vi "tls http connection handler.vi"(8 "http responder":refnum<class "http responder.lvclass">, 9 "remote address":string, 10 "basic HTTP handler dataset":refnum<class "basic HTTP handler dataset.lvclass">, 11 "connection":refnum<k5>) -> ()   [LabVIEW 2016, in "TLS HTTP server.lvclass"]
uses:
  TLS HTTP server.lvclass
  HTTP responder/http responder.lvclass
  HTTP handler dataset/basic HTTP handler dataset.lvclass
  HTTP server/http request.ctl
  HTTP server/http method.ctl
  HTTP headers/http header data.ctl
  HTTP server/http response.ctl
  HTTP server/http response packet type.ctl
  TLS handler dataset/TLS HTTP handler dataset.lvclass
  HTTP handler dataset/basic HTTP handler dataset.lvclass/basic HTTP handler dataset.ctl
  HTTP server/http parse state.ctl
  HTTP server/Basic HTTP server.lvclass
  HTTP headers/http headers.lvlib
  lvlibtls/socket connection/lvlibretls connection.lvclass
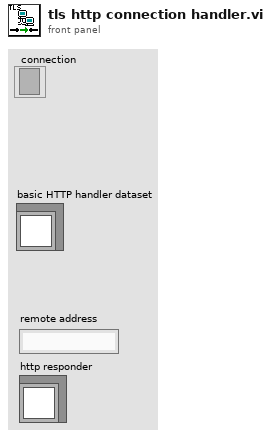
[diagram p1: front panel]
types:
  T1 = typedef "Basic HTTP server.lvclass/http response.ctl" = cluster{"packet type":T2, "reason code":u16, "status string":string, "headers":T3, "cookies":string[], "data":string}
  T2 = typedef "Basic HTTP server.lvclass/http response packet type.ctl" = enum16{"full response", "header only", "data only", "last data", "raw output"}
  T3 = typedef "http headers.lvlib/http header data.ctl" = cluster{"lookup":variant}
  T4 = typedef "Basic HTTP server.lvclass/http request.ctl" = cluster{"type":T5, "remote address":string, "method":string, "url":string, "version":string, "headers":T3, "data":string}
  T5 = typedef "Basic HTTP server.lvclass/http method.ctl" = enum16{"application", "error", "upgrade", "expect"}
  T6 = typedef "Basic HTTP server.lvclass/http server info.ctl" = cluster{"port":u16}
  T7 = typedef "Basic HTTP server.lvclass/http server properties.ctl" = cluster{"max url size":i32, "max header":i32, "timeout ms":i32, "max data size":i32}
  T8 = typedef "Basic HTTP server.lvclass/http parse state.ctl" = enum16{"function", "headers", "data"}
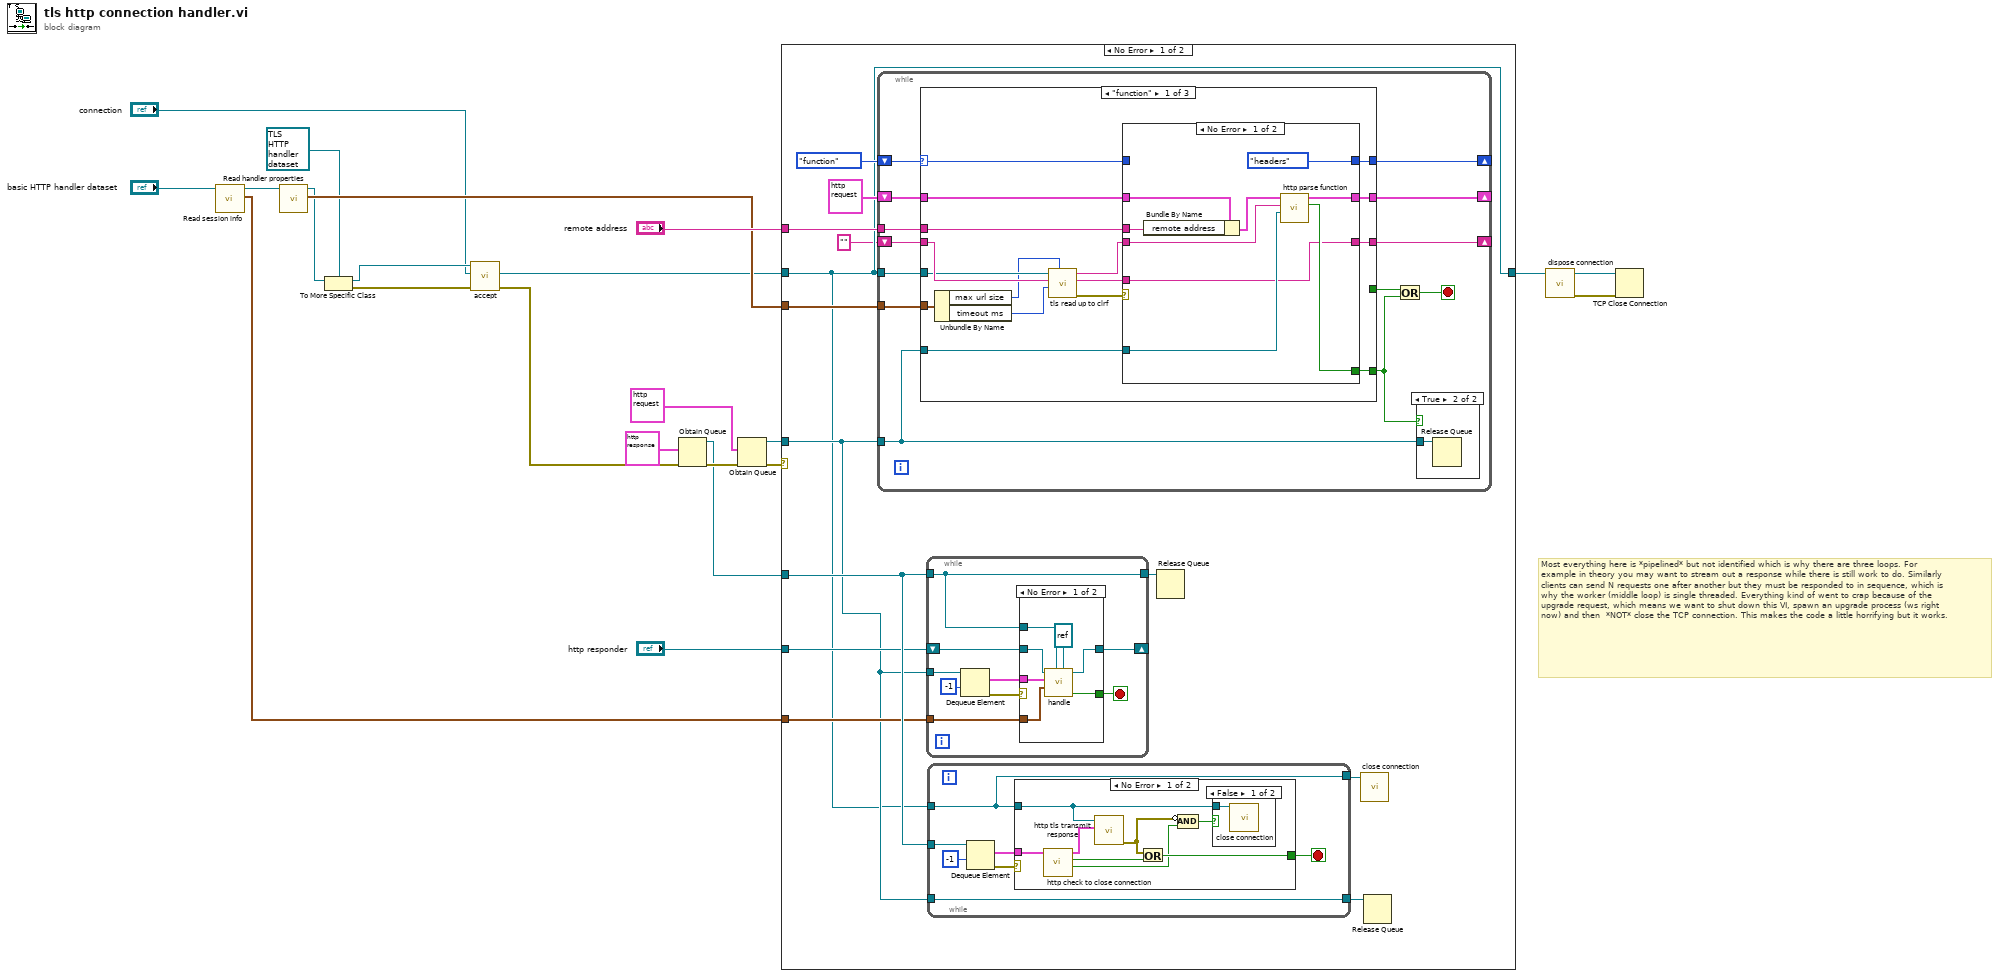
[diagram p0: block diagram]
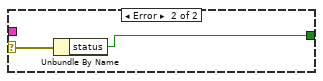
[diagram p3: hidden frame]
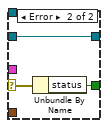
[diagram p4: hidden frame]
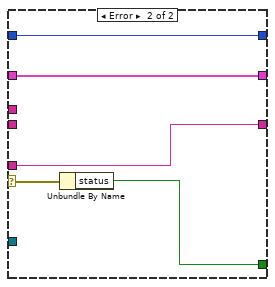
[diagram p6: hidden frame]
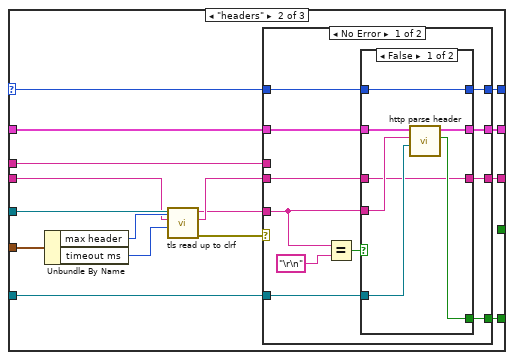
[diagram p7: hidden frame]
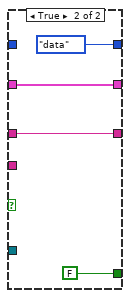
[diagram p8: hidden frame]
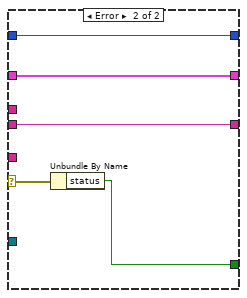
[diagram p9: hidden frame]
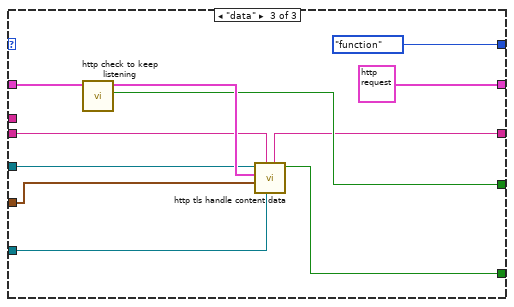
[diagram p10: hidden frame]
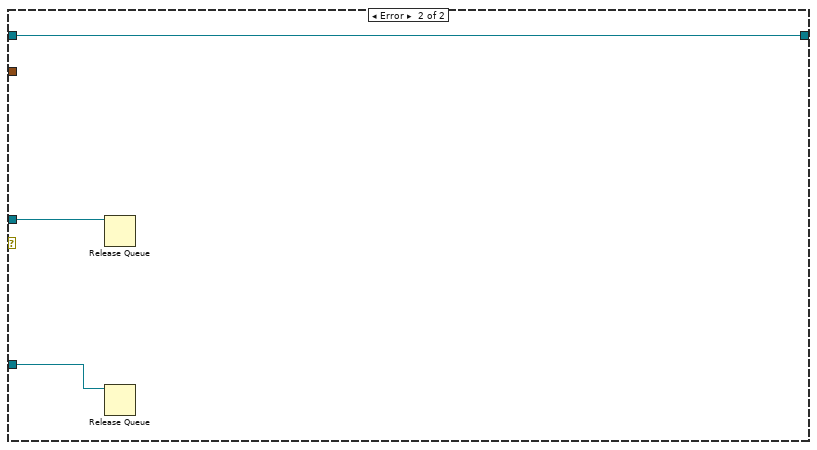
[diagram p11: hidden frame]
diagram:
  # "Most everything here is *pipelined* but not identified which is why there are three loops. For example in theory you may want to stream out a response while there is still work to do. Similarly clients can send N requests one after another but they must be responded to in sequence, which is why the worker (middle loop) is single threaded. Everything kind of went to crap because of the upgrade request, which means we want to shut down this VI, spawn an upgrade process (ws right now) and then  *NOT* close the TCP connection. This makes the code a little horrifying but it works."
  n1 = call "Read session info.vi"("basic HTTP handler dataset in"="basic HTTP handler dataset") -> ("server information"=w11:T6, "basic HTTP handler dataset out"=w13:refnum<class "basic HTTP handler dataset.lvclass">)  [unwired: 9 in]
  n2 = call "Read handler properties.vi"("basic HTTP handler dataset in"=w13) -> ("server properties"=w14:T7, "basic HTTP handler dataset out"=w10:refnum<class "basic HTTP handler dataset.lvclass">)  [unwired: 9 in]
  n3 = To More Specific Class(target class=refnum<class "TLS HTTP handler dataset.lvclass"> refnum ("TLS HTTP handler dataset"), reference=w10) -> (specific class reference=w8:refnum<class "TLS HTTP handler dataset.lvclass">, error out=w7:errorcluster)  [unwired: 1 in]
  n4 = call "accept.vi"("error in"=w7, "connection ID"="connection", "TLS HTTP handler dataset in"=w8) -> ("error out"=w6:errorcluster, "lvlibretls connection"=w5:refnum<class "lvlibretls connection.lvclass">)  [unwired: 7 in]
  n5 = Obtain Queue(element data type=T1 {"packet type"=enum."full response", "reason code"=0, "status string"="", "headers"={"lookup"=variant}, "cookies"=[], "data"=""} ("application request"), error in (no error)=w6) -> (queue out=w16:refnum<queue>, error out=w19:errorcluster)  [unwired: 3 in, 1 out]
  n6 = Obtain Queue(element data type=T4 {"type"=enum."application", "remote address"="", "method"="", "url"="", "version"="", "headers"={"lookup"=variant}, "data"=""} ("application request"), error in (no error)=w19) -> (queue out=w17:refnum<queue>, error out=w21:errorcluster)  [unwired: 3 in, 1 out]
  n7 = case shown="No Error" w21 {
    tunnel: w5 -> [w27 w171]
    tunnel: "remote address" -> [w35 _]
    tunnel: w17 -> [w29 w173]
    tunnel: w14 -> [w33 _]
    tunnel: w16 -> [w32 w172]
    tunnel: "http responder" -> [w31 _]
    tunnel: w11 -> [w30 _]
    tunnel: [w27 w171] -> w3
    frame No Error {
      n8 = while {
        tunnel: w27 -> [w75]
        shift-right: [w84] -> _
        shift-left: T4 {"type"=enum."application", "remote address"="", "method"="", "url"="", "version"="", "headers"={"lookup"=variant}, "data"=""} ("application request") -> [w85]
        tunnel: w29 -> [w77]
        shift-right: [w83] -> _
        shift-left: http_parse_state."function" -> [w80]
        tunnel: w35 -> [w82]
        tunnel: w33 -> [w81]
        shift-right: [w73] -> _
        shift-left: "" -> [w74]
        stop <- w79 stop-if-true
        n9 = case shown="\"function\"" w80 {
          selector: w80 -> [w97 w126 _]
          tunnel: w85 -> [w102 w132 w165]
          tunnel: [w101 w131 T4 {"type"=enum."application", "remote address"="", "method"="", "url"="", "version"="", "headers"={"lookup"=variant}, "data"=""} ("application request")] -> w84
          tunnel: w75 -> [w92 w121 w162]
          tunnel: [w100 w130 http_parse_state."function"] -> w83
          tunnel: [w99 w129 w168] -> w78
          tunnel: w82 -> [w98 w128 _]
          tunnel: w77 -> [w95 w127 w166]
          tunnel: w81 -> [w96 w125 w167]
          tunnel: [_ _ w163] -> w76
          tunnel: w74 -> [w94 w120 w161]
          tunnel: [w87 w124 w160] -> w73
          frame "function" {
            n10 = Unbundle By Name(w96) -> ("max url size"=w90:i32, "timeout ms"=w91:i32)
            n11 = call "tls read up to clrf.vi"("max size"=w90, "timeout ms"=w91, "buffer in"=w94, "lvlibretls connection in"=w92) -> ("error out"=w89:errorcluster, "buffer out"=w88:string, "line out"=w93:string)  [unwired: 5 in]
            n12 = case shown="No Error" w89 {
              selector: w89 -> [_ w115]
              tunnel: w102 -> [w109 w116]
              tunnel: [w110 w116] -> w101
              tunnel: [w108 w113] -> w99
              tunnel: w88 -> [w104 w112]
              tunnel: w97 -> [_ w114]
              tunnel: [http_parse_state."headers" w114] -> w100
              tunnel: w98 -> [w107 _]
              tunnel: w95 -> [w105 _]
              tunnel: w93 -> [w103 _]
              tunnel: [w104 w112] -> w87
              frame No Error {
                n13 = Bundle By Name(cluster=w109, "remote address"=w107) -> (w106:T4)
                n14 = call "http parse function.vi"("handler queue"=w105, "data in"=w103, "application request in"=w106) -> ("abort"=w108:bool, "application request out"=w110:T4)  [unwired: 7 in]
              }
              frame Error {
                n15 = Unbundle By Name(w115) -> ("status"=w113:bool)
              }
            }
          }
          frame "headers" {
            n16 = Unbundle By Name(w125) -> ("max header"=w123:i32, "timeout ms"=w122:i32)
            n17 = call "tls read up to clrf.vi"("max size"=w123, "timeout ms"=w122, "buffer in"=w120, "lvlibretls connection in"=w121) -> ("error out"=w117:errorcluster, "buffer out"=w119:string, "line out"=w118:string)  [unwired: 5 in]
            n18 = case shown="No Error" w117 {
              selector: w117 -> [_ w158]
              tunnel: w132 -> [w139 w159]
              tunnel: [w140 w159] -> w131
              tunnel: [w138 w156] -> w129
              tunnel: w127 -> [w135 _]
              tunnel: w118 -> [w142 _]
              tunnel: w126 -> [w143 w157]
              tunnel: [w141 w157] -> w130
              tunnel: w128 -> [_ _]
              tunnel: w119 -> [w133 w155]
              tunnel: [w134 w155] -> w124
              frame No Error {
                n19 = Equal?(x=w142, y="\r\n" ("x")) -> (x = y?=w136:bool)
                n20 = case shown="False" w136 {
                  tunnel: w142 -> [w149 _]
                  tunnel: w139 -> [w148 w153]
                  tunnel: [w147 w153] -> w140
                  tunnel: w143 -> [w150 _]
                  tunnel: [w150 http_parse_state."data"] -> w141
                  tunnel: [w146 FALSE ("abort")] -> w138
                  tunnel: w135 -> [w145 _]
                  tunnel: [w144 w151] -> w134
                  tunnel: w133 -> [w144 w151]
                  frame False {
                    n21 = call "http parse header.vi"("handler queue"=w145, "data in"=w149, "application request"=w148) -> ("abort"=w146:bool, "application request out"=w147:T4)  [unwired: 7 in]
                  }
                  frame True {
                  }
                }
              }
              frame Error {
                n22 = Unbundle By Name(w158) -> ("status"=w156:bool)
              }
            }
          }
          frame "data" {
            n23 = call "http check to keep listening.vi"("application request in"=w165) -> ("stop listening"=w163:bool, "application request out"=w164:T4)  [unwired: 9 in]
            n24 = call "http tls handle content data.vi"("exec queue"=w166, "buffer in"=w161, "server properties"=w167, "application request"=w164, "lvlibretls connection in"=w162) -> ("abort"=w168:bool, "buffer out"=w160:string)  [unwired: 5 in]
          }
        }
        n25 = Or(x=w76, y=w78) -> (x .or. y?=w79:bool)
        n26 = case shown="True" w78 {
          tunnel: w77 -> [_ w86]
          frame False {
          }
          frame True {
            n27 = Release Queue(queue=w86) -> ()  [unwired: 2 in, 3 out]
          }
        }
      }
      n28 = while {
        tunnel: w32 -> [w57]
        tunnel: [w57] -> w25
        tunnel: w29 -> [w62]
        shift-right: [w55] -> _
        shift-left: w31 -> [w56]
        tunnel: w30 -> [w54]
        stop <- w59 stop-if-true
        n29 = Dequeue Element(queue=w62, timeout in ms (-1)=-1) -> (element=w58:T4, error out=w60:errorcluster)  [unwired: 1 in, 2 out]
        n30 = case shown="No Error" w60 {
          selector: w60 -> [_ w72]
          tunnel: [w65 w71] -> w59
          tunnel: w58 -> [w66 _]
          tunnel: w57 -> [w69 _]
          tunnel: w56 -> [w68 w70]
          tunnel: [w67 w70] -> w55
          tunnel: w54 -> [w64 _]
          frame No Error {
            n31 = call "handle.vi"("TCP connection"=refnum<k5> refnum, "response queue"=w69, "server information"=w64, "application request in"=w66, "http responder in"=w68) -> ("stop processing"=w65:bool, "http responder out"=w67:refnum<class "http responder.lvclass">)  [unwired: 5 in]
          }
          frame Error {
            n32 = Unbundle By Name(w72) -> ("status"=w71:bool)
          }
        }
      }
      n33 = while {
        tunnel: w27 -> [w36]
        tunnel: w32 -> [w42]
        tunnel: [w37] -> w24
        tunnel: w29 -> [w37]
        tunnel: [w36] -> w23
        stop <- w39 stop-if-true
        n34 = Dequeue Element(queue=w42, timeout in ms (-1)=-1) -> (element=w38:T1, error out=w40:errorcluster)  [unwired: 1 in, 2 out]
        n35 = case shown="No Error" w40 {
          selector: w40 -> [_ w53]
          tunnel: [w46 w52] -> w39
          tunnel: w38 -> [w50 _]
          tunnel: w36 -> [w47 _]
          frame No Error {
            n36 = call "http check to close connection.vi"("application request"=w50) -> ("leave connection open?"=w44:bool, "stop process?"=w48:bool, "application request out"=w49:T1)  [unwired: 8 in]
            n37 = call "http tls transmit response.vi"("application request"=w49, "lvlibretls connection in"=w47) -> ("error out"=w43:errorcluster)  [unwired: 9 in]
            n38 = Or(x=w43, y=w48) -> (x .or. y?=w46:bool)
            n39 = Compound Arithmetic op=AND(invert w43, w44) -> (w45:bool)
            n40 = case shown="False" w45 {
              tunnel: w47 -> [w51 _]
              frame False {
                n41 = call "close connection.vi"("lvlibretls connection in"=w51) -> ()  [unwired: 9 in, 2 out]
              }
              frame True {
              }
            }
          }
          frame Error {
            n42 = Unbundle By Name(w53) -> ("status"=w52:bool)
          }
        }
      }
      n43 = Release Queue(queue=w25) -> ()  [unwired: 2 in, 3 out]
      n44 = call "close connection.vi"("lvlibretls connection in"=w23) -> ()  [unwired: 9 in, 2 out]
      n45 = Release Queue(queue=w24) -> ()  [unwired: 2 in, 3 out]
    }
    frame Error {
      n46 = Release Queue(queue=w173) -> ()  [unwired: 2 in, 3 out]
      n47 = Release Queue(queue=w172) -> ()  [unwired: 2 in, 3 out]
    }
  }
  n48 = call "dispose connection.vi"("lvlibretls connection in"=w3) -> ("error out"=w1:errorcluster, "connection"=w2:refnum<k5>)  [unwired: 9 in]
  n49 = TCP Close Connection(connection ID=w2, error in (no error)=w1) -> ()  [unwired: 1 in, 2 out]
